vi "Periodic Tasks.vi"(8 "error in":errorcluster) -> ()   [LabVIEW 2017]
doc: "This VI runs in parallel to other robot code. It can contain as many user-defined periodic loops as you need. These can carry out PID or other sorts of timed response."
uses:
  <vilib>/Rock Robotics/Network Tables/NT Read Boolean.vi
  <vilib>/Rock Robotics/Network Tables/NT Read String.vi
  <vilib>/Rock Robotics/Network Tables/NT Write String.vi
  <vilib>/Rock Robotics/Network Tables/NT Write String Array.vi
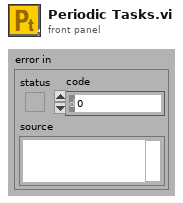
[diagram p1: front panel]
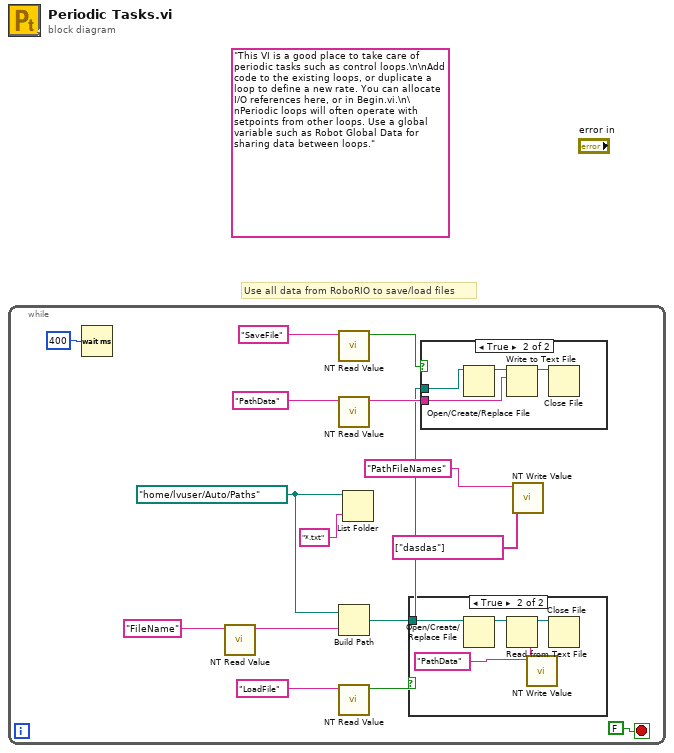
[diagram p0: block diagram]
diagram:
  (unwired) "This VI is a good place to take care of periodic tasks such as control loops.\n\nAdd code to the existing loops, or duplicate a loop to define a new rate. You can allocate I/O references here, or in Begin.vi.\n\nPeriodic loops will often operate with setpoints from other loops. Use a global variable such as Robot Global Data for sharing data between loops."
  # "Use all data from RoboRIO to save/load files"
  n1 = while {
    stop <- FALSE stop-if-true
    w3 = path "/home/lvuser/Auto/Paths" ("base path")
    n2 = Wait (ms)(milliseconds to wait=u32 400) -> ()  [unwired: 1 out]
    n3 = call-poly <vilib>:"NT Read Value.vi"("Name"="FileName") -> ("String"=w6:string)  [unwired: 9 in, 1 out]
    n4 = call-poly <vilib>:"NT Read Value.vi"("Name"="SaveFile") -> ("Boolean"=w2:bool)  [unwired: 9 in, 1 out]
    n5 = call-poly <vilib>:"NT Read Value.vi"("Name"="PathData") -> ("String"=w9:string)  [unwired: 9 in, 1 out]
    n6 = Build Path(base path=w3, name or relative path=w6) -> (appended path=w5:path)
    n7 = call-poly <vilib>:"NT Read Value.vi"("Name"="LoadFile") -> ("Boolean"=w13:bool)  [unwired: 9 in, 1 out]
    n8 = List Folder(path=w3, pattern="*.txt") -> ()  [unwired: 2 in, 4 out]
    n9 = case shown="True" w13 {
      tunnel: w5 -> [_ w18]
      frame False {
      }
      frame True {
        n10 = Open/Create/Replace File(file path (use dialog)=w18) -> (refnum out=w20:refnum<file>)  [unwired: 5 in, 2 out]
        n11 = Read from Text File(file (use dialog)=w20) -> (refnum out=w19:refnum<file>, text=w16:string)  [unwired: 3 in, 2 out]
        n12 = call-poly <vilib>:"NT Write Value.vi"("String"=w16, "Name"="PathData") -> ()  [unwired: 9 in, 1 out]
        n13 = Close File(refnum=w19) -> ()  [unwired: 1 in, 2 out]
      }
    }
    n14 = case shown="True" w2 {
      tunnel: w9 -> [_ w22]
      tunnel: w5 -> [_ w21]
      frame False {
      }
      frame True {
        n15 = Open/Create/Replace File(file path (use dialog)=w21) -> (refnum out=w24:refnum<file>)  [unwired: 5 in, 2 out]
        n16 = Write to Text File(file (use dialog)=w24, text=w22) -> (refnum out=w23:refnum<file>)  [unwired: 2 in, 2 out]
        n17 = Close File(refnum=w23) -> ()  [unwired: 1 in, 2 out]
      }
    }
    n18 = call-poly <vilib>:"NT Write Value.vi"("String Array"=string[] ["dasdas"], "Name"="PathFileNames") -> ()  [unwired: 9 in, 1 out]
  }
